vi "Read Project Refnum.vi"(8 "error in (no error)":errorcluster, 11 "Test Runner.Project in":refnum<class "Test Runner.Project.lvclass">) -> (0 "error out":errorcluster, 2 "Project Refnum":refnum<vi>, 3 "Test Runner.Project out":refnum<class "Test Runner.Project.lvclass">)   [LabVIEW 2013, in "Caraya.lvlib" / "Test Runner.Project.lvclass"]
uses:
  Test Runner.Project.lvclass
  Test Runner.Project.lvclass/Test Runner.Project.ctl
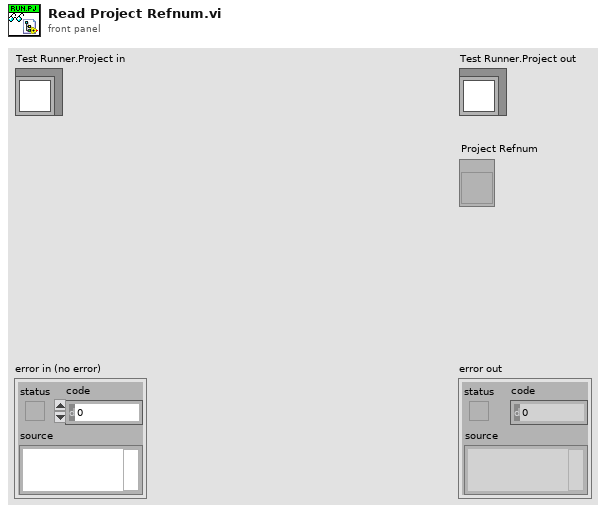
[diagram p1: front panel]
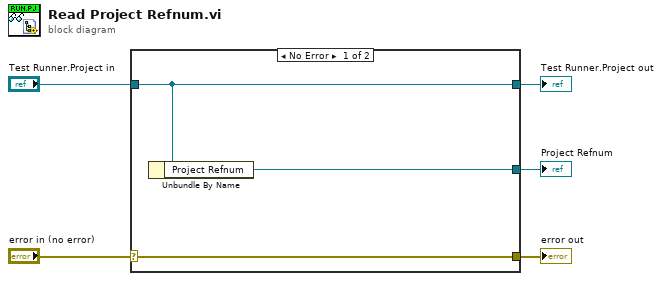
[diagram p0: block diagram]
diagram:
  n1 = case shown="No Error" "error in (no error)" {
    selector: "error in (no error)" -> [w8 w9]
    tunnel: [w8 w9] -> w4
    tunnel: [w7 w10] -> w2
    tunnel: "Test Runner.Project in" -> [w7 w10]
    tunnel: [w6 _] -> w1
    frame No Error {
      n2 = Unbundle By Name(w7) -> ("Project Refnum"=w6:refnum<vi>)
    }
    frame Error {
    }
  }
  "error out" <- w4
  "Test Runner.Project out" <- w2
  "Project Refnum" <- w1
